vi "SLSC Ask to Erase Configuration.vi"(8 "error in (no error)":errorcluster, 10 "Ask to erase?":bool, 11 "Device Item Ref in":T1 format="%.0x") -> (0 "error out":errorcluster, 1 "Erase Data?":bool, 2 "initialized?":bool, 3 "Item Ref out":T1 format="%.0x")   [LabVIEW 2019, in "SLSC EDS System Explorer.lvlib"]
uses:
  SLSC EDS System Explorer.lvlib
  <vilib>/NI VeriStand/Custom Device API/Custom Device Item Ref.ctl
  Shared/Constants.vi
  <vilib>/NI VeriStand/Custom Device API/Get Item Property (Boolean).vi
  <vilib>/NI VeriStand/Custom Device API/Custom Device API.lvlib
  Shared/SLSC EDS Shared.lvlib
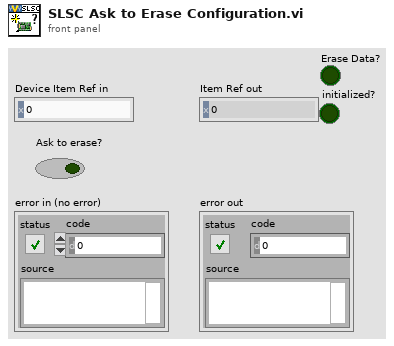
[diagram p1: front panel]
types:
  T1 = typedef "Custom Device API.lvlib/Custom Device Item Ref.ctl" = u64
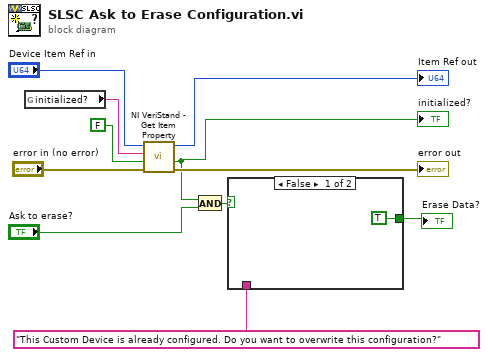
[diagram p0: block diagram]
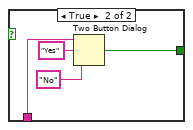
[diagram p2: hidden frame]
diagram:
  n1 = global read "Constants.vi" "initialized?"() -> (w7:string)
  n2 = call-poly <vilib>:"NI VeriStand - Get Item Property.vi"("error in (no error)"="error in (no error)", "Default Value"=FALSE, "Property Name"=w7, "Item Ref in"="Device Item Ref in") -> ("error out"=→"error out":errorcluster, "Value"=w5:bool, "Item Ref out"=→"Item Ref out":T1)  [unwired: 4 in, 1 out]
  "initialized?" <- w5
  n3 = And(x=w5, y="Ask to erase?") -> (x .and. y?=w2:bool)
  n4 = case shown="False" w2 {
    tunnel: "This Custom Device is already configured. Do you want to overwrite this configuration?" ("message") -> [_ w16]
    tunnel: [TRUE ("T button?") w13] -> w1
    frame False {
    }
    frame True {
      n5 = Two Button Dialog(message=w16, 1:"No" ("F button name (\"Cancel\")"), 2:"Yes" ("T button name (\"OK\")")) -> (T button?=w13:bool)
    }
  }
  "Erase Data?" <- w1
